vi "AES-Cipher-text.vi"(5 "Initializer Vector":string, 7 "Operation Mode":T1, 8 "error in (no error)":errorcluster, 9 "cipher [U8]":u8[](array[numeric]), 10 "Cipher Key":string, 11 "Message in":string) -> (0 "error out":errorcluster, 1 "cipher out":u8[](array[numeric]), 3 "Ciphered message":string)   [LabVIEW 2020, in "Encryption.lvlib"]
doc: "Encripts the <b>text<b> in using the cipher and the given <b>Operation Mode</b>.\nCAUTION:\nThis VI is not secure, it does not protect the memory of the encryption, key and unencrypted data.\n\n(c) Ton Plomp, 2011\nTHIS SOFTWARE IS PROVIDED AS IS, AND ANY WARRANTY IS REJECTED"
uses:
  Encryption.lvlib
  AES-Modes.ctl
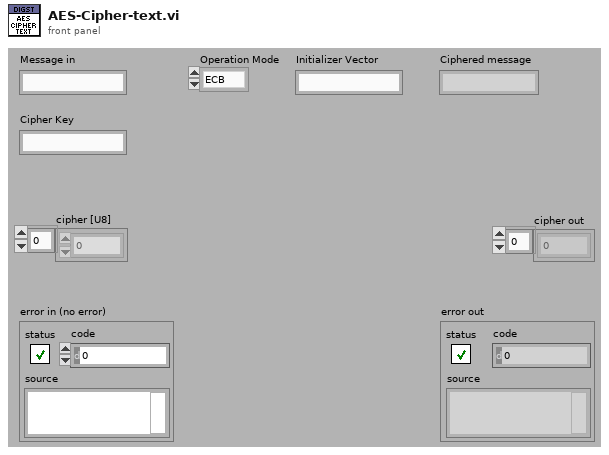
[diagram p1: front panel]
types:
  T1 = typedef "Encryption.lvlib/AES-Modes.ctl" = enum16{"ECB", "CBC", "CFB128", "OFB"}
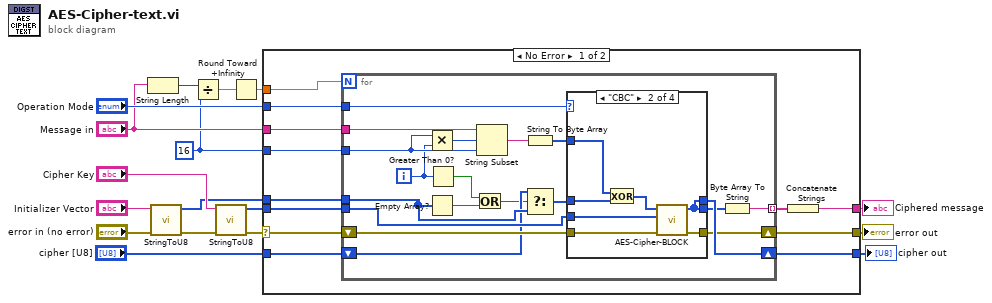
[diagram p0: block diagram]
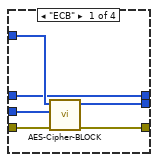
[diagram p2: hidden frame]
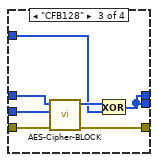
[diagram p3: hidden frame]
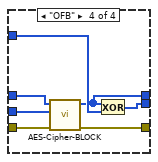
[diagram p4: hidden frame]
diagram:
  w3 = 16 ("y")
  n1 = String Length(string="Message in") -> (length=w4:i32)
  n2 = call "StringToU8.vi"("error in (no error)"="error in (no error)", "HEX text in"="Initializer Vector") -> ("error out"=w10:errorcluster, "ArrayU8 out"=w8:u8[])  [unwired: 8 in]
  n3 = Divide(x=w4, y=w3) -> (x/y=w6:dbl)
  n4 = call "StringToU8.vi"("error in (no error)"=w10, "HEX text in"="Cipher Key") -> ("error out"=w15:errorcluster, "ArrayU8 out"=w14:u8[])  [unwired: 8 in]
  n5 = Round Toward +Infinity(x=w6) -> (ceil(x): smallest int >= x=w5:dbl)
  n6 = case shown="No Error" w15 {
    selector: w15 -> [w25 w77]
    tunnel: "Message in" -> [w29 _]
    tunnel: [w24 w77] -> w17
    tunnel: w14 -> [w28 _]
    tunnel: w5 -> [w27 _]
    tunnel: w3 -> [w26 _]
    tunnel: [w22 _] -> w13
    tunnel: "Operation Mode" -> [w21 _]
    tunnel: w8 -> [w20 _]
    tunnel: "cipher [U8]" -> [w19 w76]
    tunnel: [w18 w76] -> w1
    frame No Error {
      n7 = for {
        N: w27 -> [_]
        tunnel: w29 -> [w40]
        tunnel: w28 -> [w48]
        tunnel: w26 -> [w46]
        shift-right: [w32] -> w24
        shift-left: w25 -> [w43]
        tunnel: [w31] -> w23 mode=indexing
        tunnel: w21 -> [w42]
        shift-right: [w41] -> w18
        shift-left: w19 -> [w37]
        tunnel: w20 -> [w39]
        i -> [w35]
        n8 = Multiply(x=w46, y=w35) -> (x*y=w47:i32)
        n9 = Empty Array?(array=w39) -> (empty?=w34:bool)
        n10 = Greater Than 0?(x=w35) -> (x > 0?=w36:bool)
        n11 = Or(x=w36, y=w34) -> (x .or. y?=w33:bool)
        n12 = String Subset(string=w40, offset (0)=w47, length (rest)=w46) -> (substring=w45:string)
        n13 = String To Byte Array(string=w45) -> (unsigned byte array=w44:u8[])
        n14 = Select(t=w37, s=w33, f=w39) -> (s? t:f=w38:u8[])
        n15 = case shown="\"CBC\"" w42 {
          tunnel: w48 -> [w54 w61 w68 w75]
          tunnel: w44 -> [w53 w55 w63 w71]
          tunnel: w43 -> [w52 w60 w67 w74]
          tunnel: [w51 w57 w62 w70] -> w30
          tunnel: [w50 w59 w66 w73] -> w32
          tunnel: w38 -> [w49 w58 w65 w72]
          tunnel: [w49 w57 w62 w69] -> w41
          frame "ECB" {
            n16 = call "AES-Cipher-BLOCK.vi"("error in (no error)"=w52, "Cipher Key"=w54, "Plain [U8]"=w53) -> ("error out"=w50:errorcluster, "cipher [U8]"=w51:u8[])  [unwired: 7 in]
          }
          frame "CBC" {
            n17 = Exclusive Or(1:w58, 2:w55) -> (0:w56:u8[])
            n18 = call "AES-Cipher-BLOCK.vi"("error in (no error)"=w60, "Cipher Key"=w61, "Plain [U8]"=w56) -> ("error out"=w59:errorcluster, "cipher [U8]"=w57:u8[])  [unwired: 7 in]
          }
          frame "CFB128" {
            n19 = call "AES-Cipher-BLOCK.vi"("error in (no error)"=w67, "Cipher Key"=w68, "Plain [U8]"=w65) -> ("error out"=w66:errorcluster, "cipher [U8]"=w64:u8[])  [unwired: 7 in]
            n20 = Exclusive Or(1:w63, 2:w64) -> (0:w62:u8[])
          }
          frame "OFB" {
            n21 = call "AES-Cipher-BLOCK.vi"("error in (no error)"=w74, "Cipher Key"=w75, "Plain [U8]"=w72) -> ("error out"=w73:errorcluster, "cipher [U8]"=w69:u8[])  [unwired: 7 in]
            n22 = Exclusive Or(1:w71, 2:w69) -> (0:w70:u8[])
          }
        }
        n23 = Byte Array To String(unsigned byte array=w30) -> (string=w31:string)
      }
      n24 = Concatenate Strings(w23) -> (w22:string)
    }
    frame Error {
    }
  }
  "error out" <- w17
  "Ciphered message" <- w13
  "cipher out" <- w1
